vi "PlayAlarm.vi"(2 "Alarm Button":bool) -> ()   [LabVIEW 2020]
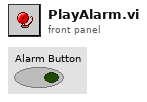
[diagram p1: front panel]
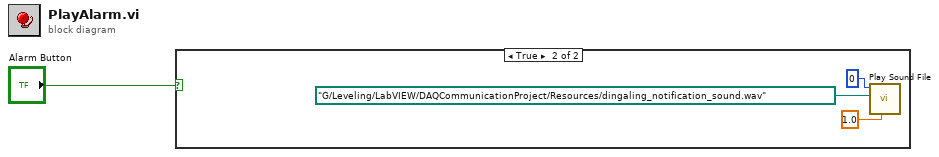
[diagram p0: block diagram]
diagram:
  n1 = case shown="True" "Alarm Button" {
    frame False {
    }
    frame True {
      n2 = call <vilib>:"Play Sound File.vi"("timeout (sec)"=1.0, "path"=path "G:/Leveling/LabVIEW/DAQCommunicationProject/Resources/dingaling_notification_sound.wav", "device ID"=u32 0) -> ()  [unwired: 7 in, 2 out]
    }
  }
